vi "User Console.vi"(8 "error in (no error)":errorcluster, 11 "Seq Context":refnum<k7>) -> (0 "error out":errorcluster)   [LabVIEW 2021, in "User Console.lvlib"]
uses:
  User Console.lvlib
  Private Controls/Images.ctl
  Private Controls/Local Variable.ctl
  User Event/UE Control.ctl
  User Event/UE Dataset.ctl
  <vilib>/addons/TestStand/_TSUtility.llb/TestStand - Start Modal Dialog (Sequence Context).vi
  <vilib>/addons/TestStand/_TSUtility.llb/TestStand - End Modal Dialog (Sequence Context).vi
  User Event/User Event.lvlib
  Controller/EOL Controller.lvlib
panel:
  in  "Image Filename":T1 items=["DMM Expand.jpg", "ACIR Expand.jpg", "DMM Retract.jpg", "ACIR Retract.jpg", "Retract All.jpg"]
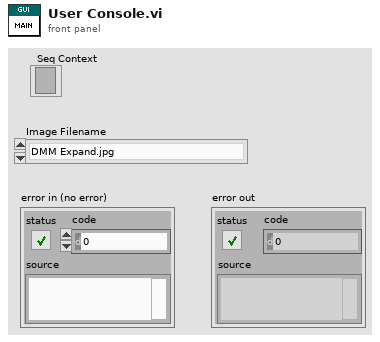
[diagram p1: front panel]
types:
  T1 = typedef "User Console.lvlib/Images.ctl" = u16
  T2 = typedef "User Console.lvlib/Local Variable.ctl" = cluster{"Sequence Context":refnum<k7>, "Image Filename":refnum<vi>, "Modal ID":i32, "Image path":path, "This VI":refnum<vi>}
  T3 = typedef "User Event.lvlib/UE Dataset.ctl" = cluster{"Message":string, "Data":variant}
  T4 = typedef "User Event.lvlib/UE Control.ctl" = enum16{"Create", "Get", "Generate", "Destroy"}
  T5 = typedef "User Console.lvlib/Module Action.ctl" = enum16{"Init", "Error", "Close", "Select Test", "Start Test"}
  T6 = typedef "Images.ctl" = u16
  T7 = typedef "imagedata.ctl" = cluster{"image type":i32, "image depth":i32, "image":u8[], "mask":u8[], "colors":u32[], "Rectangle":cluster{"left":i16, "top":i16, "right":i16, "bottom":i16}}
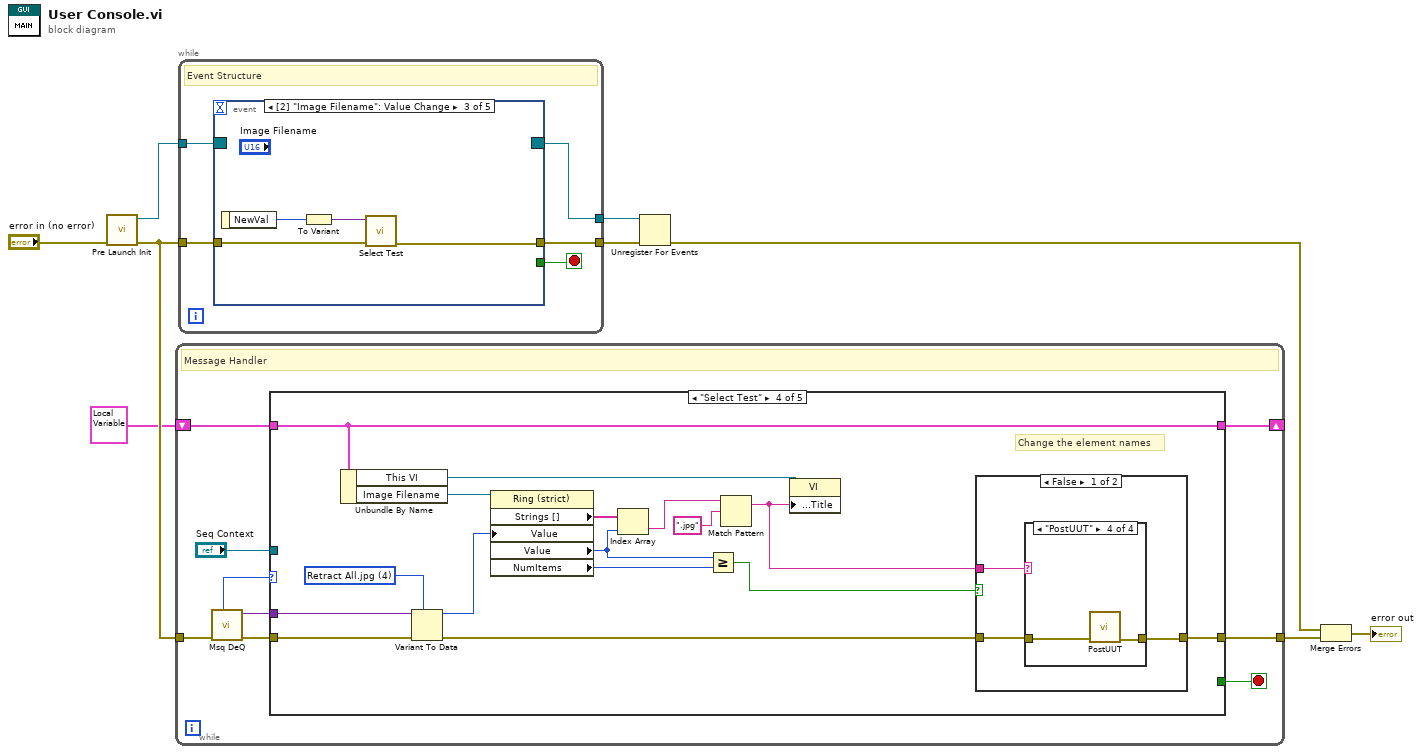
[diagram p0: block diagram]
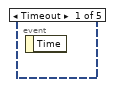
[diagram p2: hidden frame]
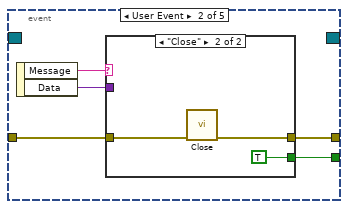
[diagram p3: hidden frame]
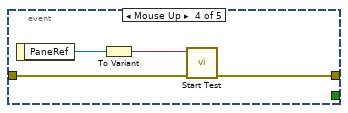
[diagram p5: hidden frame]
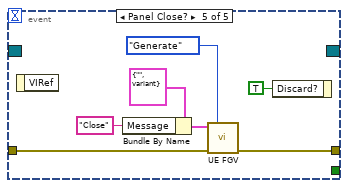
[diagram p6: hidden frame]
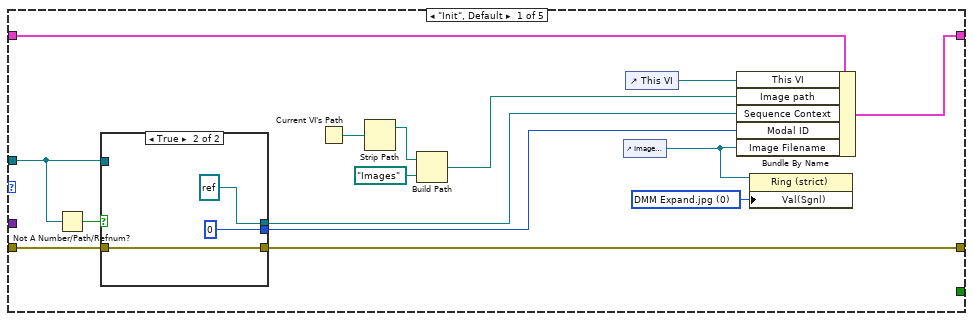
[diagram p7: hidden frame]
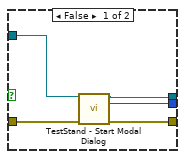
[diagram p8: hidden frame]
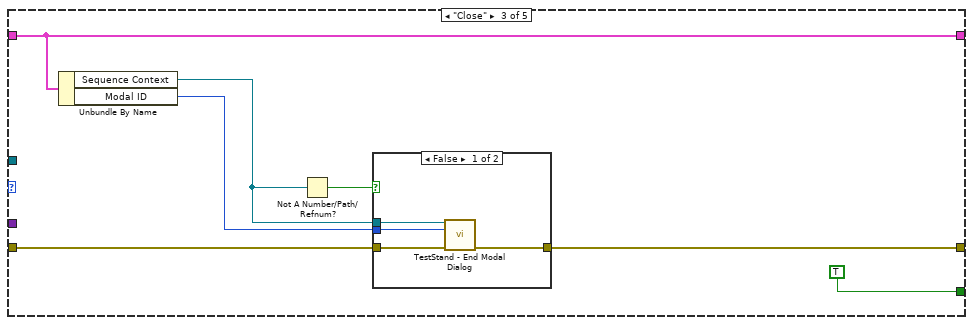
[diagram p10: hidden frame]
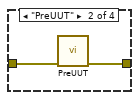
[diagram p13: hidden frame]
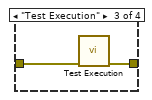
[diagram p14: hidden frame]
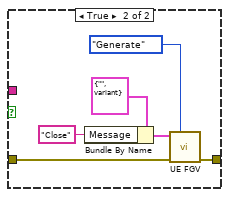
[diagram p15: hidden frame]
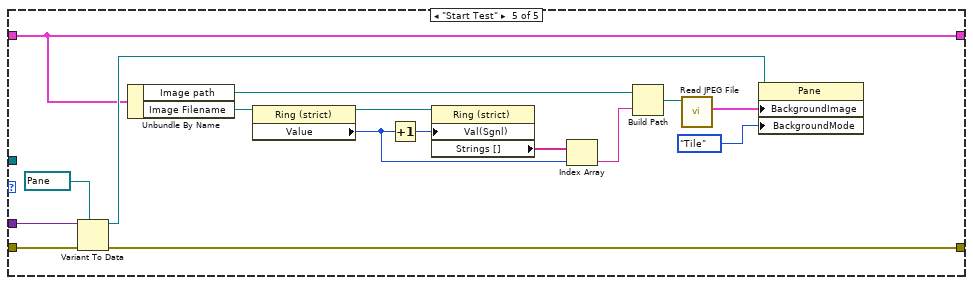
[diagram p16: hidden frame]
diagram:
  n1 = call "Pre Launch Init.vi"("error in (no error)"="error in (no error)") -> ("error out"=w3:errorcluster, "Event Registration Refnum"=w8:refnum<event-registration>)  [unwired: 9 in]
  n2 = while {
    tunnel: w3 -> [w18]
    tunnel: [w13] -> w2
    shift-right: [w10] -> _
    shift-left: T2 {"Sequence Context"=refnum, "Image Filename"=refnum, "Modal ID"=0, "Image path"=path "", "This VI"=refnum} ("Cluster") -> [w11]
    stop <- w14 stop-if-true
    # "Message Handler"
    n3 = call "Msq DeQ.vi"("error in (no error)"=w18) -> ("error out"=w16:errorcluster, "Data"=w15:variant, "Module Action"=w17:T5)  [unwired: 8 in]
    n4 = case shown="\"Select Test\"" w17 {
      tunnel: w16 -> [w31 _ w47 w68 w102]
      tunnel: w15 -> [_ _ _ w67 w101]
      tunnel: [_ _ TRUE _ _] -> w14
      tunnel: [w22 _ w45 w62 w88] -> w13
      tunnel: "Seq Context" -> [w32 _ _ _ _]
      tunnel: w11 -> [w30 w42 w48 w70 w87]
      tunnel: [w27 w42 w48 w70 w87] -> w10
      frame "Init", Default {
        w25 = T1 0 items=["DMM Expand.jpg", "ACIR Expand.jpg", "DMM Retract.jpg", "ACIR Retract.jpg", "Retract All.jpg"] ("Value (Signaling)")
        n5 = Not A Number/Path/Refnum?(number/path/refnum=w32) -> (NaN/Path/Refnum?=w33:bool)
        n6 = case shown="True" w33 {
          tunnel: w31 -> [w37 w41]
          tunnel: [w36 w41] -> w22
          tunnel: w32 -> [w38 _]
          tunnel: [w35 refnum<k7> refnum ("Sequence Context Out")] -> w29
          tunnel: [w34 0 ("Modal ID")] -> w28
          frame False {
            n7 = call-poly <vilib>:"TestStand - Start Modal Dialog.vi"("Sequence Context In"=w38, "error in (no error)"=w37) -> ("Sequence Context Out"=w35:refnum<k7>, "Modal ID"=w34:i32, "error out"=w36:errorcluster)  [unwired: 9 in, 2 out]
          }
          frame True {
          }
        }
        n8 = Current VI's Path() -> (path=w20:path)
        n9 = Strip Path(path=w20) -> (stripped path=w19:path)  [unwired: 1 out]
        n10 = Build Path(base path=w19, name or relative path=path "Images") -> (appended path=w23:path)
        n11 = control-ref of="Image Filename"() -> (w26:refnum<vi>)
        n12 = control-ref of="This VI"() -> (w21:refnum<vi>)
        n13 = Bundle By Name(cluster=w30, "This VI"=w21, "Image path"=w23, "Sequence Context"=w29, "Modal ID"=w28, "Image Filename"=w26) -> (w27:T2)
        n14 = property class="Ring (strict)"(reference=w26, "Val(Sgnl)"=w25) -> ()  [unwired: 1 in, 2 out]
      }
      frame "Error" {
      }
      frame "Close" {
        n15 = Unbundle By Name(w48) -> ("Sequence Context"=w44:refnum<k7>, "Modal ID"=w46:i32)
        n16 = Not A Number/Path/Refnum?(number/path/refnum=w44) -> (NaN/Path/Refnum?=w43:bool)
        n17 = case shown="False" w43 {
          tunnel: w47 -> [w53 w54]
          tunnel: w46 -> [w52 _]
          tunnel: [w51 w54] -> w45
          tunnel: w44 -> [w50 _]
          frame False {
            n18 = call-poly <vilib>:"TestStand - End Modal Dialog.vi"("Sequence Context In"=w50, "Modal ID"=w52, "error in (no error)"=w53) -> ("error out"=w51:errorcluster)  [unwired: 12 in]
          }
          frame True {
          }
        }
      }
      frame "Select Test" {
        w66 = T1 4 items=["DMM Expand.jpg", "ACIR Expand.jpg", "DMM Retract.jpg", "ACIR Retract.jpg", "Retract All.jpg"] ("Ring")
        # "Change the element names"
        n19 = Unbundle By Name(w70) -> ("This VI"=w60:refnum<vi>, "Image Filename"=w69:refnum<vi>)
        n20 = Variant To Data(error in=w68, type=w66, Variant=w67) -> (data=w59:T1, error out=w55:errorcluster)
        n21 = property class="Ring (strict)"(reference=w69, "Value"=w59) -> ("Strings []"=w63:string[], "Value"=w58:T6, "NumItems"=w65:u32)  [unwired: 1 in, 2 out]
        n22 = Index Array(array=w63, index=w58) -> (element=w57:string)
        n23 = Greater Or Equal?(x=w58, y=w65) -> (x >= y?=w61:bool)
        n24 = Match Pattern(string=w57, regular expression=".jpg") -> (before substring=w56:string)  [unwired: 1 in, 3 out]
        n25 = property class="VI"(reference=w60, "Front Panel.Title"=w56) -> ()  [unwired: 1 in, 2 out]
        n26 = case shown="False" w61 {
          tunnel: [w71 w86] -> w62
          tunnel: w55 -> [w72 w81]
          tunnel: w56 -> [w73 _]
          frame False {
            n27 = case shown="\"PostUUT\"" w73 {
              tunnel: w72 -> [w74 w76 w78 w80]
              tunnel: [w74 w75 w77 w79] -> w71
              frame Default {
              }
              frame "PreUUT" {
                n28 = call "PreUUT.vi"("error in (no error)"=w76) -> ("error out"=w75:errorcluster)  [unwired: 10 in]
              }
              frame "Test Execution" {
                n29 = call "Test Execution.vi"("error in (no error)"=w78) -> ("error out"=w77:errorcluster)  [unwired: 10 in]
              }
              frame "PostUUT" {
                n30 = call "PostUUT.vi"("error in (no error)"=w80) -> ("error out"=w79:errorcluster)  [unwired: 10 in]
              }
            }
          }
          frame True {
            n31 = Bundle By Name(cluster=T3 {"Message"="", "Data"=variant} ("event data"), "Message"="Close") -> (w84:T3)
            n32 = call "UE FGV.vi"("UE Ctls"=UE_Control."Generate", "error in (no error)"=w81, "event data"=w84) -> ("error out"=w86:errorcluster)  [unwired: 7 in, 1 out]
          }
        }
      }
      frame "Start Test" {
        n33 = Variant To Data(error in=w102, type=refnum<vi> refnum ("PaneRef"), Variant=w101) -> (data=w95:refnum<vi>, error out=w88:errorcluster)
        n34 = Unbundle By Name(w87) -> ("Image path"=w94:path, "Image Filename"=w99:refnum<vi>)
        n35 = property class="Ring (strict)"(reference=w99) -> (reference out=w90:refnum<vi>, "Value"=w91:T6)  [unwired: 1 in, 1 out]
        n36 = Increment(x=w91) -> (x+1=w92:T6)
        n37 = property class="Ring (strict)"(reference=w90, "Val(Sgnl)"=w92) -> ("Strings []"=w93:string[])  [unwired: 1 in, 2 out]
        n38 = Index Array(array=w93, index=w91) -> (element=w89:string)
        n39 = Build Path(base path=w94, name or relative path=w89) -> (appended path=w98:path)
        n40 = call <vilib>:"Read JPEG File.vi"("path to JPEG file"=w98) -> ("image data"=w96:T7)  [unwired: 8 in, 2 out]
        n41 = property class="Pane"(reference=w95, "BackgroundImage"=w96, "BackgroundMode"=enum16{"Stretch", "Center", "Tile"}."Tile" ("Background Mode")) -> ()  [unwired: 1 in, 2 out]
      }
    }
  }
  n42 = while {
    tunnel: w3 -> [w106]
    tunnel: w8 -> [w107]
    tunnel: [w104] -> w7
    tunnel: [w103] -> w6
    stop <- w105 stop-if-true
    # "Event Structure"
    n43 = event shown="[2] \"Image Filename\": Value Change" {
      selector: w107 -> [_ _ _ _ _]
      dyn-events: [_ _ _ _ _] -> w103
      timeout: _ -> [_ _ _ _ _]
      tunnel: w106 -> [_ w110 w120 w124 w126]
      tunnel: [_ w109 w119 w123 w125] -> w104
      tunnel: [_ w108 _ _ _] -> w105
      event Timeout {
        n44 = event-data() -> ()  [unwired: 1 in, 1 out]
      }
      event User Event {
        n45 = event-data() -> ("Message"=w112:string, "Data"=w111:variant)  [unwired: 1 in]
        n46 = case shown="\"Close\"" w112 {
          tunnel: w111 -> [_ _]
          tunnel: w110 -> [w113 w116]
          tunnel: [w113 w115] -> w109
          tunnel: [_ TRUE] -> w108
          frame Default {
          }
          frame "Close" {
            n47 = call "Close.vi"("error in (no error)"=w116) -> ("error out"=w115:errorcluster)  [unwired: 10 in]
          }
        }
      }
      event Value Change {
        n48 = event-data() -> ("NewVal"=w118:T1)  [unwired: 1 in]
        n49 = To Variant(anything=w118) -> (Variant=w117:variant)
        n50 = call "Select Test.vi"("error in (no error)"=w120, "Data"=w117) -> ("error out"=w119:errorcluster)  [unwired: 9 in]
      }
      event Mouse Up {
        n51 = event-data() -> ("PaneRef"=w122:refnum<vi>)  [unwired: 1 in]
        n52 = To Variant(anything=w122) -> (Variant=w121:variant)
        n53 = call "Start Test.vi"("error in (no error)"=w124, "Data"=w121) -> ("error out"=w123:errorcluster)  [unwired: 9 in]
      }
      event Panel Close? {
        n54 = event-data() -> ()  [unwired: 1 in, 1 out]
        n55 = Bundle By Name(cluster=T3 {"Message"="", "Data"=variant} ("event data"), "Message"="Close") -> (w128:T3)
        n56 = call "UE FGV.vi"("UE Ctls"=UE_Control."Generate", "error in (no error)"=w126, "event data"=w128) -> ("error out"=w125:errorcluster)  [unwired: 7 in, 1 out]
        n57 = event-data("Discard?"=TRUE) -> ()  [unwired: 1 in, 1 out]
      }
    }
  }
  n58 = Unregister For Events(event registration refnum=w6, error in=w7) -> (error out=w5:errorcluster)
  n59 = Merge Errors(w5, w2) -> (→"error out":errorcluster)
